vi "PDC_GetTriggerMode.vi"(0 "DeviceNo":u32, 11 "error in (no error)":errorcluster) -> (3 "Mode":u32, 4 "ReturnValue":u32, 6 "AFrames":u32, 8 "RFrames":u32, 10 "RCount":u32, 14 "ErrorCode":u32, 15 "error out":errorcluster)   [LabVIEW 2015]
doc: "This VI retrieves the trigger mode of the specified device."
uses:
  PDCLIB.dll
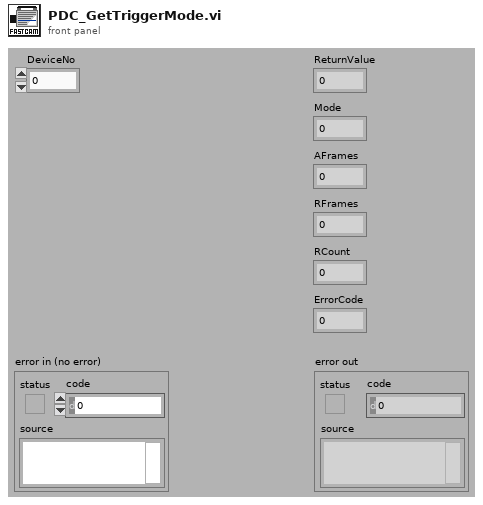
[diagram p1: front panel]
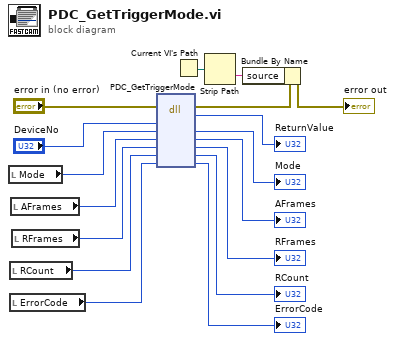
[diagram p0: block diagram]
diagram:
  n1 = local read "Mode"() -> (w11:u32)
  n2 = local read "RCount"() -> (w6:u32)
  n3 = local read "ErrorCode"() -> (w14:u32)
  n4 = local read "AFrames"() -> (w10:u32)
  n5 = local read "RFrames"() -> (w7:u32)
  n6 = dll-call lib="PDCLIB.dll" fn="PDC_GetTriggerMode"(error in="error in (no error)", "nDeviceNo"="DeviceNo", "pMode"=w11, "pAFrames"=w10, "pRFrames"=w7, "pRCount"=w6, "pErrorCode"=w14) -> (error out=w2:errorcluster, "return type"=→"ReturnValue":u32, "pMode"=→"Mode":u32, "pAFrames"=→"AFrames":u32, "pRFrames"=→"RFrames":u32, "pRCount"=→"RCount":u32, "pErrorCode"=→"ErrorCode":u32)  [unwired: 3 in, 1 out]
  n7 = Current VI's Path() -> (path=w3:path)
  n8 = Strip Path(path=w3) -> (name=w4:string)  [unwired: 1 out]
  n9 = Bundle By Name(cluster=w2, "source"=w4) -> (→"error out":errorcluster)
